vi "CV_Measurements.vi"() -> ()   [LabVIEW 2017]
uses:
  <vilib>/Utility/file.llb/Write Delimited Spreadsheet (DBL).vi
  Program Files/National Instruments/LabVIEW 2017/instr.lib/Agilent E4980/Agilent E4980.lvlib
  <vilib>/Analysis/NI_AALPro.lvlib
panel:
  in  "secret":bool caption="OK Button"
  out "Steps":dbl
  out "Q":dbl
  in  "stop":bool
  in  "Save":bool
  out "Width (mm)":dbl
  out "Capacitance (pF)":dbl
  out "NW":cluster{dbl[], ext[unit][]}(graph) caption="Primary"
  out "1_C2V":cluster{dbl[], dbl[]}(graph)={[-1.0], [1.8568866883502444e+20]} caption="Primary"
  in  "Save to:":path=path "C:/Users/Noah/Desktop/CV_test.txt"
  out "CV":cluster{dbl[], dbl[]}(graph)={[-1.0], [73.385]} caption="Primary"
  in  "error in (no error)":errorcluster
  in  "Manual Impedance Range (3: 100 Ohms) 2":i32(ring)=3 items=["100m", "1", "10", "100", "300", "1K", "3K", "10K", "30K", "100K"]
  in  "VISA resource name":refnum<visa-resource-name>="USB0::0x0957::0x0909::MY46101893::INSTR"
  in  "Relative Permittivity, er":dbl=1.044 caption="Permittivity (pF/cm)"
  in  "Signal Frequency (kHz)":dbl=1000.0
  in  "Voltage Increment (V)":dbl=0.05
  in  "Final Voltage (V)":dbl=3.0
  in  "Initial Voltage (V)":dbl=0.1
  in  "Area (cm^2)":dbl=0.005153 format="%#_6e"
  in  "Enable Auto Range (T:Enable) 2":bool=TRUE
  in  "Signal Type (0: Voltage) 2":u16(ring) items=["Voltage"]
  in  "Function (0: Cp-D) 2":u16(ring)=1 items=["Cp-D", "Cp-Q", "Cp-G", "Cp-Rp", "Cs-D", "Cs-Q", "Cs-Rs", "Lp-D", "Lp-Q", "Lp-G", "Lp-Rp", "Lp-Rdc", "Ls-D", "Ls-Q", "Ls-Rs", "Ls-Rdc", "R-X", "Z-thd", "Z-thr", "G-B", "Y-thd", "Y-thr", "Vdc-Idc"]
  # "e0 = 0.088542 pF/cm"
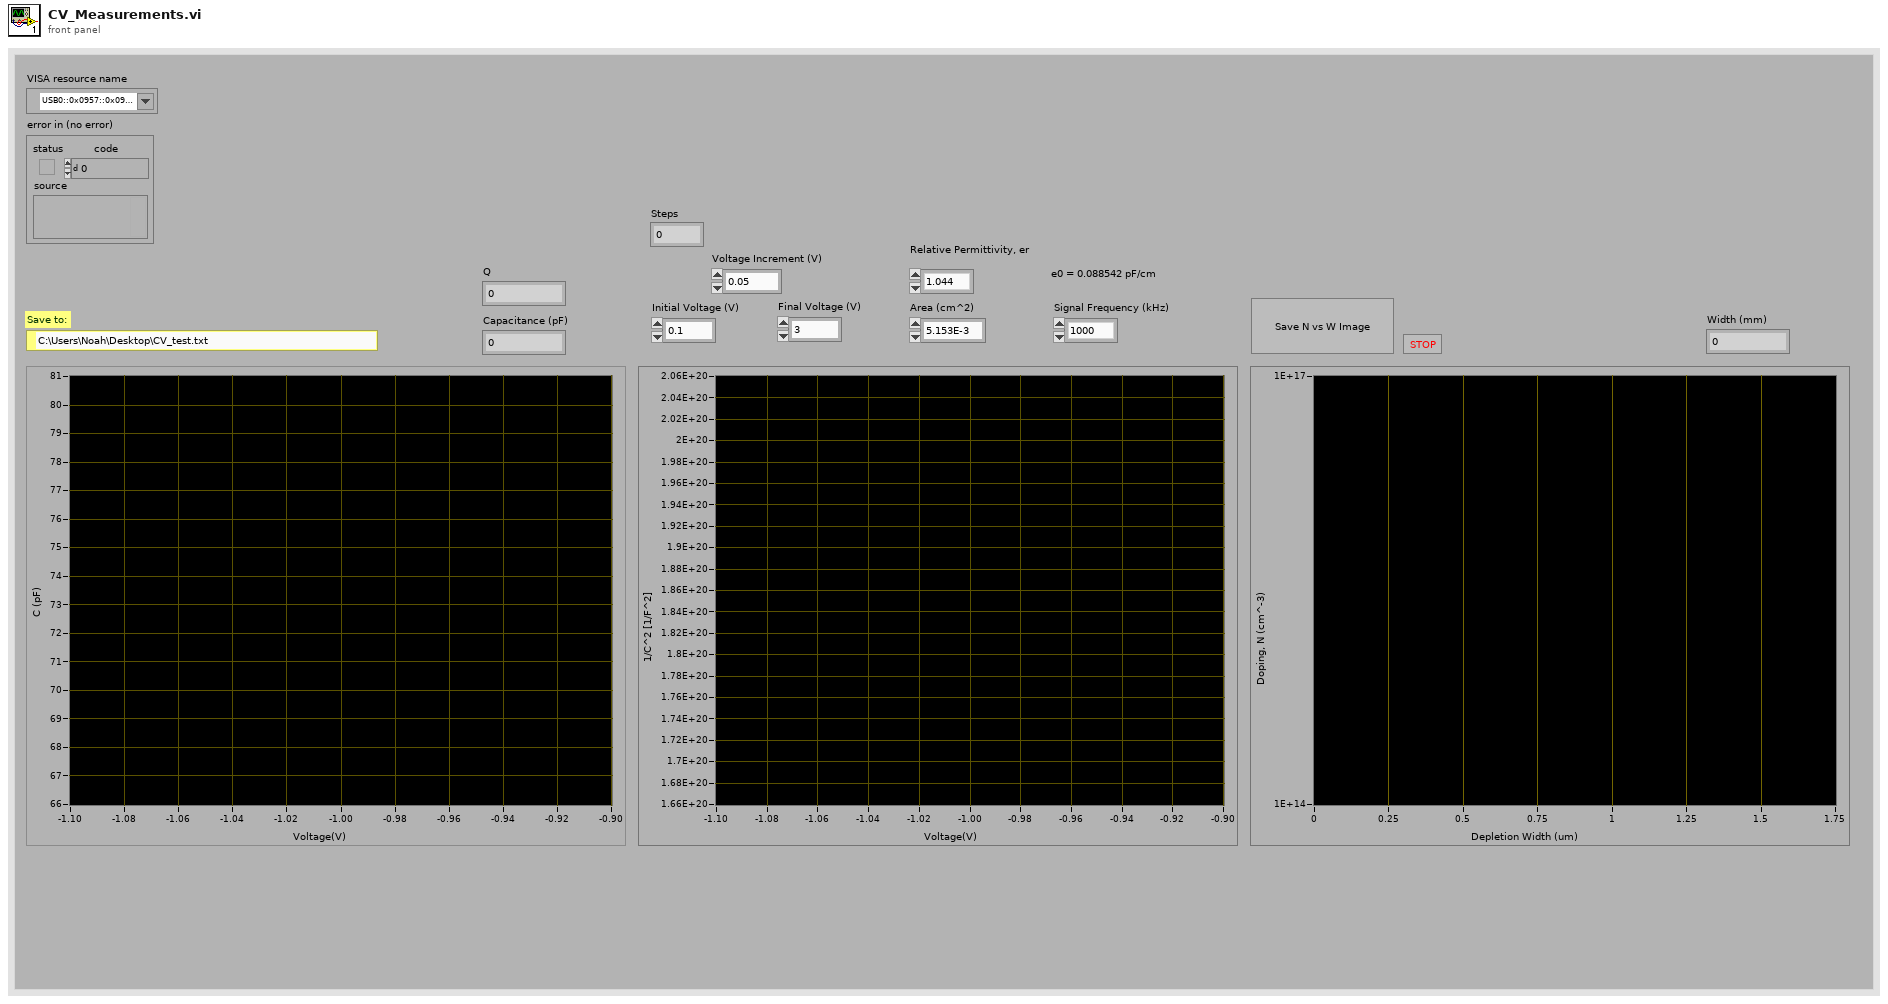
[diagram p1: front panel]
types:
  T1 = typedef "imagedata.ctl" = cluster{"image type":i32, "image depth":i32, "image":u8[], "mask":u8[], "colors":u32[], "Rectangle":cluster{"left":i16, "top":i16, "right":i16, "bottom":i16}}
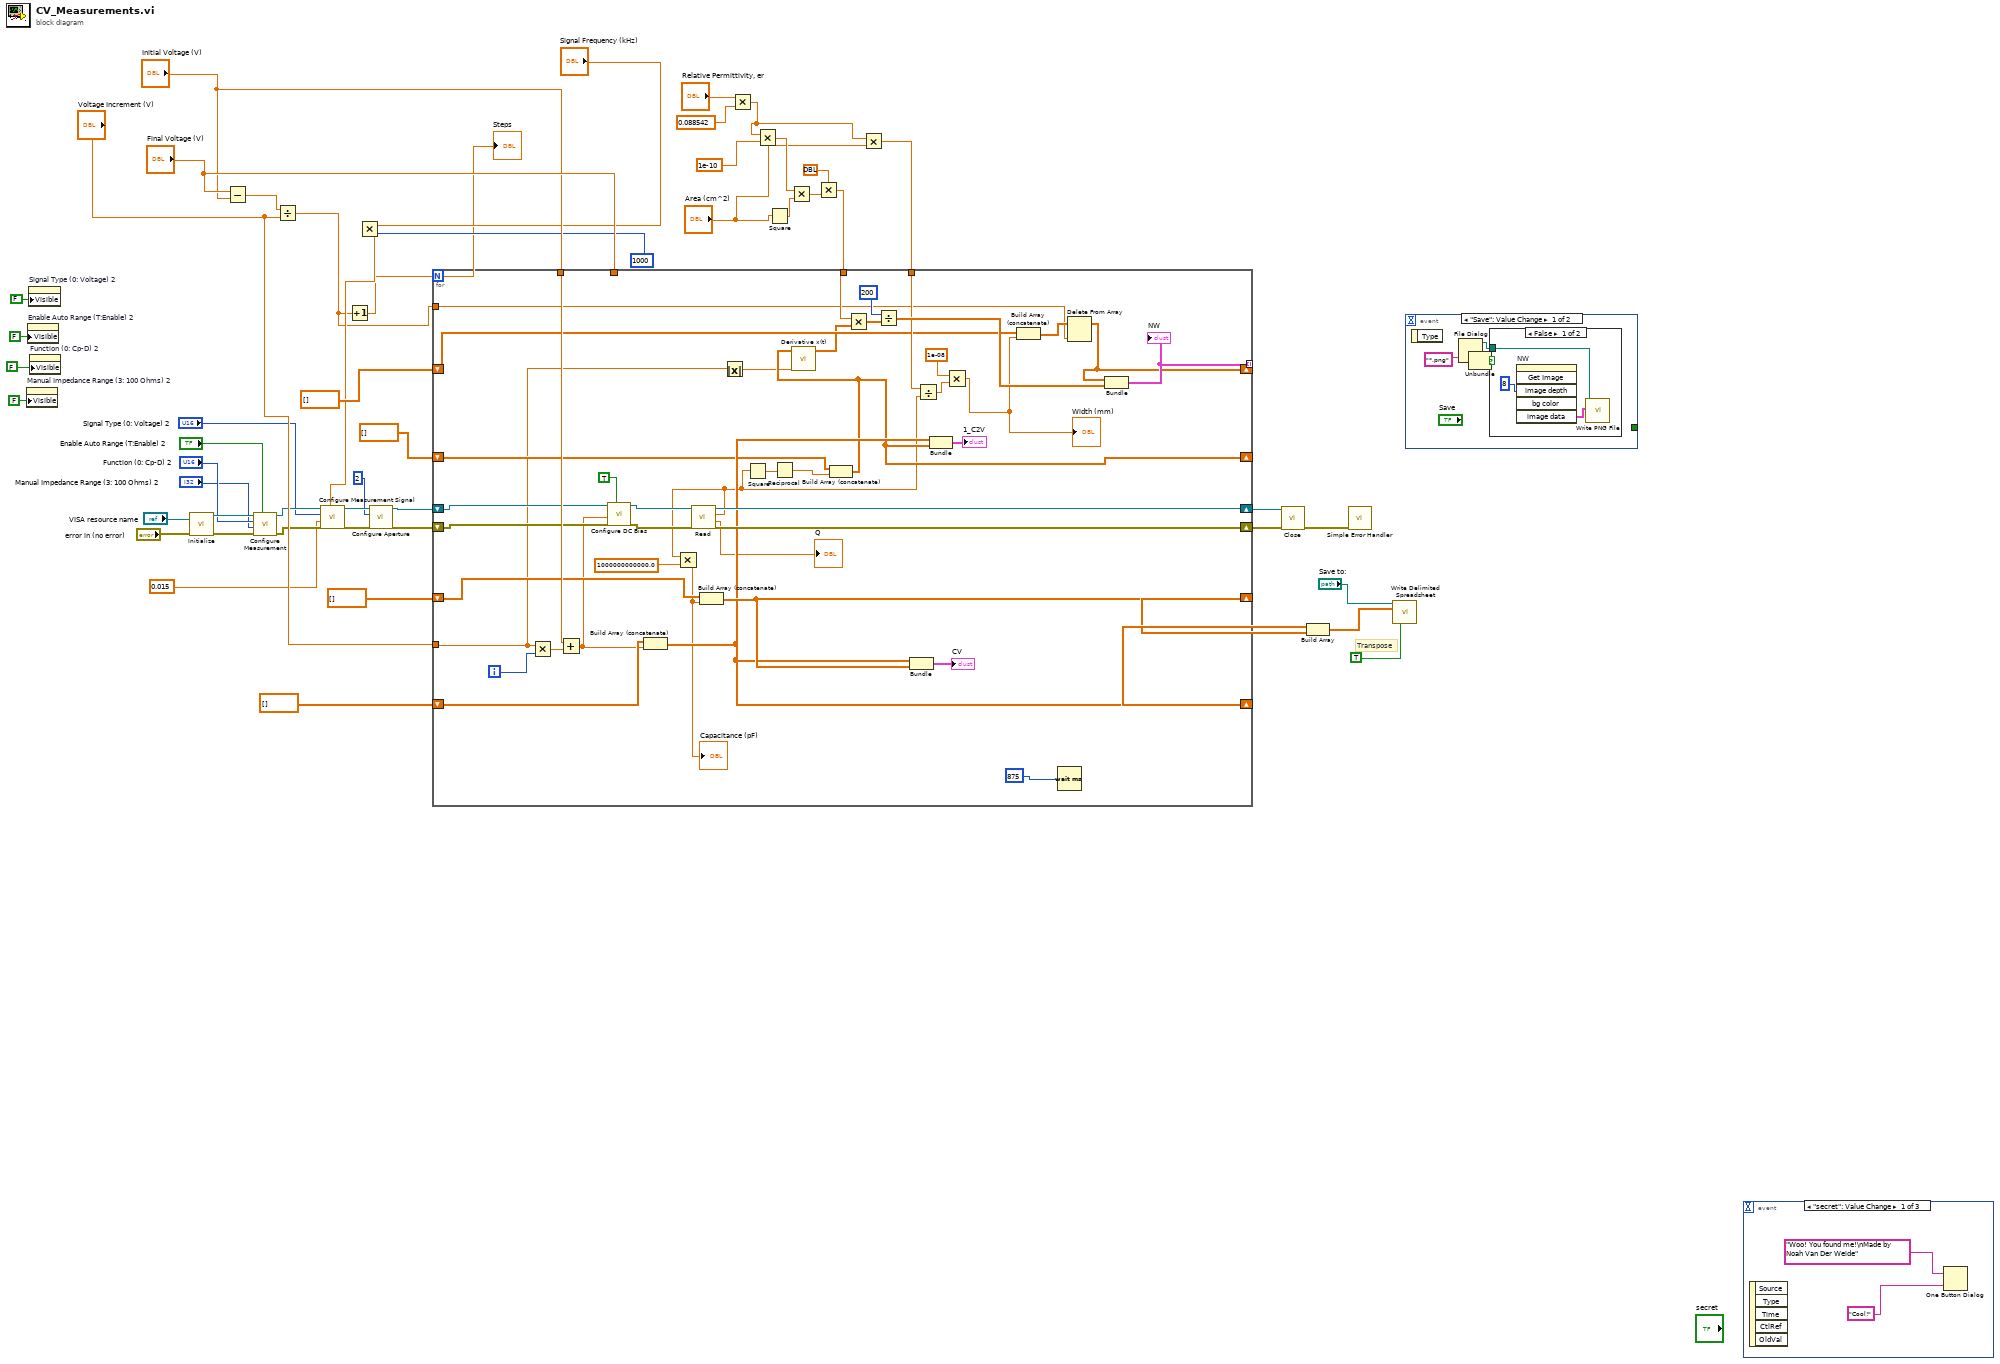
[diagram p0: block diagram]
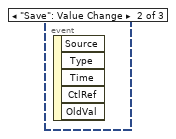
[diagram p2: hidden frame]
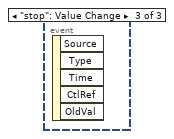
[diagram p3: hidden frame]
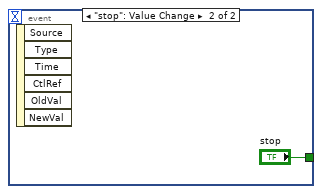
[diagram p5: hidden frame]
diagram:
  # "Transpose"
  n1 = property on="Manual Impedance Range (3: 100 Ohms) 2" class="Ring (strict)"("Visible"=FALSE) -> ()  [unwired: 2 in, 2 out]
  n2 = property on="Enable Auto Range (T:Enable) 2" class="Bool (strict)"("Visible"=FALSE) -> ()  [unwired: 2 in, 2 out]
  n3 = property on="Signal Type (0: Voltage) 2" class="Ring (strict)"("Visible"=FALSE) -> ()  [unwired: 2 in, 2 out]
  n4 = property on="Function (0: Cp-D) 2" class="Ring (strict)"("Visible"=FALSE) -> ()  [unwired: 2 in, 2 out]
  n5 = call "Initialize.vi"("error in (no error)"="error in (no error)", "VISA resource name"="VISA resource name") -> ("error out"=w46:errorcluster, "VISA resource name out"=w47:refnum<visa-resource-name>)  [unwired: 8 in]
  n6 = Subtract(x="Final Voltage (V)", y="Initial Voltage (V)") -> (x-y=w51:dbl)
  n7 = call "Configure Measurement.vi"("Enable Auto Range (T:Enable)"="Enable Auto Range (T:Enable) 2", "error in (no error)"=w46, "Manual Impedance Range (3: 100 Ohms)"="Manual Impedance Range (3: 100 Ohms) 2", "Function (0: Cp-D)"="Function (0: Cp-D) 2", "VISA resource name"=w47) -> ("error out"=w19:errorcluster, "VISA resource name out"=w18:refnum<visa-resource-name>)  [unwired: 5 in]
  n8 = Divide(x=w51, y="Voltage Increment (V)") -> (x/y=w5:dbl)
  n9 = Increment(x=w5) -> (x+1=w6:dbl)
  "Steps" <- w6
  n10 = Multiply(x="Signal Frequency (kHz)", y=1000) -> (x*y=w16:dbl)
  n11 = call "Configure Measurement Signal.vi"("Signal Frequency (1000 Hz)"=w16, "error in (no error)"=w19, "Signal Level (1.0 V)"=0.015, "Signal Type (0: Voltage)"="Signal Type (0: Voltage) 2", "VISA resource name"=w18) -> ("error out"=w14:errorcluster, "VISA resource name out"=w13:refnum<visa-resource-name>)  [unwired: 5 in]
  n12 = call "Configure Aperture.vi"("error in (no error)"=w14, "Measurement Time (1: Medium)"=2, "VISA resource name"=w13) -> ("error out"=w10:errorcluster, "VISA resource name out"=w11:refnum<visa-resource-name>)  [unwired: 7 in]
  n13 = Multiply(x="Relative Permittivity, er", y=0.088542) -> (x*y=w7:dbl)
  n14 = Multiply(x=w7, y=1e-10) -> (x*y=w27:dbl)
  n15 = Square(x="Area (cm^2)") -> (x^2=w32:dbl)
  n16 = Multiply(x=w27, y=w32) -> (x*y=w31:dbl)
  n17 = Multiply(x=ext[unit] 1.6021766208e-19, y=w31) -> (x*y=w30:ext[unit])
  n18 = Multiply(x=w7, y="Area (cm^2)") -> (x*y=w26:dbl)
  n19 = for {
    N: w6 -> [_]
    tunnel: "Voltage Increment (V)" -> [w58]
    tunnel: "Final Voltage (V)" -> [_]
    tunnel: "Initial Voltage (V)" -> [w82]
    shift-right: [w76] -> w33
    shift-left: dbl[] [] -> [w94]
    shift-right: [w81] -> w25
    shift-left: dbl[] [] -> [w75]
    tunnel: w30 -> [w88]
    tunnel: w26 -> [w79]
    shift-right: [w60] -> _
    shift-left: dbl[] [] -> [w73]
    shift-right: [w61] -> _
    shift-left: dbl[] [] -> [w64]
    tunnel: [w72] -> _ mode=indexing
    shift-right: [w92] -> w36
    shift-left: w10 -> [w70]
    shift-right: [w78] -> w37
    shift-left: w11 -> [w71]
    tunnel: w5 -> [w62]
    i -> [w84]
    n20 = Multiply(x=w58, y=w84) -> (x*y=w83:dbl)
    n21 = Add(x=w82, y=w83) -> (x+y=w67:dbl)
    n22 = call "Configure DC Bias.vi"("DC Bias State (F:Disable)"=TRUE, "error in (no error)"=w70, "DC Bias Level (0.0 V)"=w67, "VISA resource name"=w71) -> ("error out"=w69:errorcluster, "VISA resource name out"=w68:refnum<visa-resource-name>)  [unwired: 6 in]
    n23 = Build Array (concatenate)(w94, w67) -> (w76:dbl[])
    n24 = call "Read.vi"("error in (no error)"=w69, "VISA resource name"=w68) -> ("error out"=w92:errorcluster, "Secondary Parameter"=→"Q":dbl, "Primary Parameter"=w54:dbl, "VISA resource name out"=w78:refnum<visa-resource-name>)  [unwired: 6 in]
    n25 = Multiply(x=w54, y=1000000000000.0) -> (x*y=w74:dbl)
    "Capacitance (pF)" <- w74
    n26 = Build Array (concatenate)(w75, w74) -> (w81:dbl[])
    n27 = Absolute Value(x=w58) -> (abs(x)=w57:dbl)
    n28 = Square(x=w54) -> (x^2=w90:dbl)
    n29 = Reciprocal(x=w90) -> (1/x=w77:dbl)
    n30 = Build Array (concatenate)(w73, w77) -> (w60:dbl[])
    n31 = call <vilib>:"Derivative x(t).vi"("dt"=w57, "X"=w60) -> ("dX/dt"=w59:dbl[])  [unwired: 8 in, 1 out]
    n32 = Multiply(x=w88, y=w59) -> (x*y=w87:ext[unit][])
    n33 = Divide(x=200, y=w87) -> (x/y=w86:ext[unit][])
    n34 = Bundle(w76, w81) -> (→"CV":cluster{dbl[], dbl[]})  [unwired: 1 out]
    n35 = Divide(x=w79, y=w54) -> (x/y=w56:dbl)
    n36 = Bundle(w76, w60) -> (→"1_C2V":cluster{dbl[], dbl[]})  [unwired: 1 out]
    n37 = Multiply(x=1e-08, y=w56) -> (x*y=w53:dbl)
    "Width (mm)" <- w53
    n38 = Build Array (concatenate)(w64, w53) -> (w63:dbl[])
    n39 = Wait (ms)(milliseconds to wait=875) -> ()  [unwired: 1 out]
    n40 = Delete From Array(array=w63, index=w62) -> (array with subset deleted=w61:dbl[])  [unwired: 1 in, 1 out]
    n41 = Bundle(w61, w86) -> (w72:cluster{dbl[], ext[unit][]})  [unwired: 1 out]
    "NW" <- w72
  }
  n42 = call "Close.vi"("error in (no error)"=w36, "VISA resource name"=w37) -> ("error out"=w38:errorcluster)  [unwired: 9 in]
  n43 = Build Array(w33, w25) -> (w39:dbl[][])
  n44 = call <vilib>:"Simple Error Handler.vi"("error in (no error)"=w38) -> ()  [unwired: 4 in, 5 out]
  n45 = call-poly <vilib>:"Write Delimited Spreadsheet.vi"("file path (dialog if empty)"="Save to:", "2D data"=w39, "transpose? (no:F)"=TRUE) -> ()  [unwired: 11 in, 2 out]
  n46 = event shown="[0] \"Save\": Value Change" {
    selector: _ -> [_ _]
    dyn-events: _ -> [_ _]
    timeout: _ -> [_ _]
    tunnel: [_ "stop"] -> _
    event "Save": Value Change {
      n47 = event-data() -> ()  [unwired: 1 in, 1 out]
      n48 = File Dialog(6:"*.png" ("pattern")) -> (0:w95:errorcluster, 1:w97:bool, 3:w98:path)  [unwired: 6 in, 1 out]
      n49 = Unbundle(w95) -> ()  [unwired: 3 out]
      n50 = case shown="False" w97 {
        tunnel: w98 -> [w101 _]
        frame False {
          n51 = invoke on="NW" class="XYGraph (strict)" method="Get Image"("image depth"=8) -> ("image data"=w99:T1)  [unwired: 5 in, 5 out]
          n52 = call <vilib>:"Write PNG File.vi"("image data"=w99, "path to PNG file"=w101) -> ()  [unwired: 8 in, 2 out]
        }
        frame True {
        }
      }
    }
    event "stop": Value Change {
      n53 = event-data() -> ()  [unwired: 1 in, 6 out]
    }
  }
  n54 = event shown="[0] \"secret\": Value Change" {
    selector: _ -> [_ _ _]
    dyn-events: _ -> [_ _ _]
    timeout: _ -> [_ _ _]
    event "secret": Value Change {
      n55 = event-data() -> ()  [unwired: 1 in, 5 out]
      n56 = One Button Dialog(message="Woo! You found me!\nMade by Noah Van Der Weide", button name ("OK")="Cool!") -> ()  [unwired: 1 out]
    }
    event "Save": Value Change {
      n57 = event-data() -> ()  [unwired: 1 in, 5 out]
    }
    event "stop": Value Change {
      n58 = event-data() -> ()  [unwired: 1 in, 5 out]
    }
  }
